vi "写输出状态.vi"(8 "error in (no error)":errorcluster, 9 "value":bool, 10 "通道":enum16{"通道0", "通道1", "通道2", "通道3"}(ring), 11 "MB session in":refnum<class "MB_Master.lvclass">) -> (0 "error out":errorcluster, 3 "MB session out":refnum<class "MB_Master.lvclass">)   [LabVIEW 2016, in "DAM395CF.lvlib"]
uses:
  DAM395CF.lvlib
  <vilib>/Plasmionique/MB Master/MB_Master/MB_Master.lvclass
  <vilib>/Plasmionique/MB Master/MB Master.lvlib
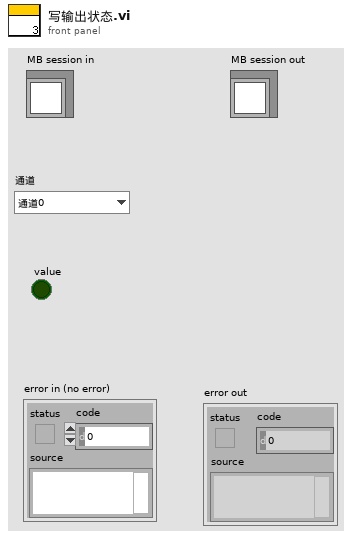
[diagram p1: front panel]
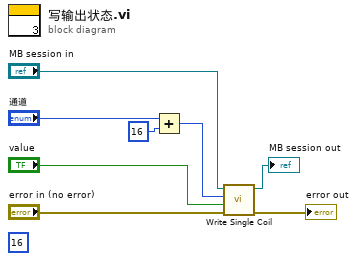
[diagram p0: block diagram]
diagram:
  (unwired) u16 16 ("starting address")
  n1 = Add(x="通道", y=16) -> (x+y=w2:i32)
  n2 = call <vilib>:"Write Single Coil.vi"("error in (no error)"="error in (no error)", "value"="value", "address"=w2, "MB session in"="MB session in") -> ("error out"=→"error out":errorcluster, "MB session out"=→"MB session out":refnum<class "MB_Master.lvclass">)  [unwired: 6 in]
